vi "Add Expected Heartbeat.vi"(6 "Timeout":u16 format="%d ms", 8 "error in":errorcluster, 9 "Period":u16 format="%d ms", 10 "Node-ID":u8, 11 "CANopen Master in":refnum<class "CANopen Master.lvclass">) -> (0 "error out":errorcluster, 3 "CANopen Master out":refnum<class "CANopen Master.lvclass">)   [LabVIEW 2024, in "CANopen Master.lvlib" / "CANopen Master.lvclass"]
uses:
  CANopen Master.lvclass
  CANopen Master.lvclass/CANopen Master.ctl
  Network Management/Network Mangement.lvclass
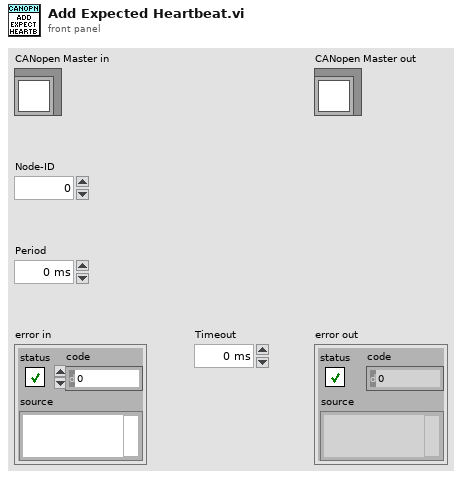
[diagram p1: front panel]
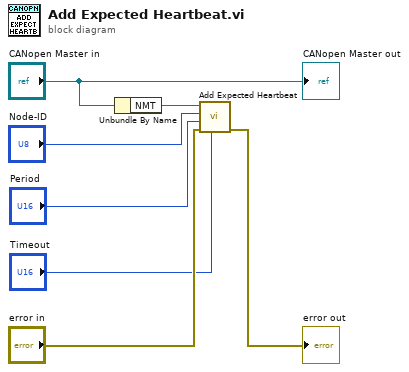
[diagram p0: block diagram]
diagram:
  n1 = Unbundle By Name("CANopen Master in") -> ("NMT"=w4:refnum<class "Network Mangement.lvclass">)
  n2 = call-dynamic "Add Expected Heartbeat.vi"("Timeout"="Timeout", "error in"="error in", "Period"="Period", "Node-ID"="Node-ID", "Network Mangement in"=w4) -> ("error out"=→"error out":errorcluster)  [unwired: 5 in, 1 out]
  "CANopen Master out" <- "CANopen Master in"
